vi "2-Sine Wave Chart (while loop with property nodes).vi"() -> ()   [LabVIEW 2014]
panel:
  in  "Color Box":u32(colorbox)
  in  "stop":bool
  out "Waveform Chart":dbl(graph)
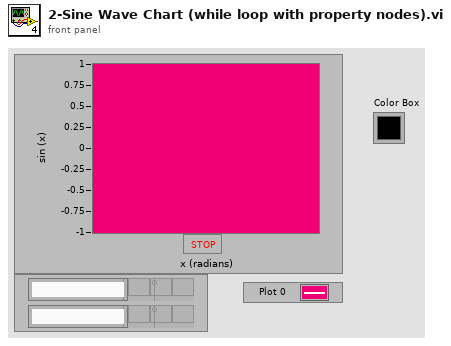
[diagram p1: front panel]
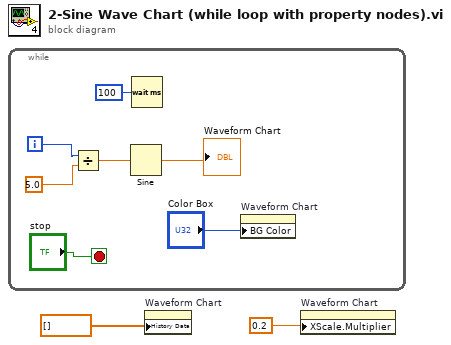
[diagram p0: block diagram]
diagram:
  n1 = while {
    i -> [w5]
    stop <- "stop" stop-if-true
    n2 = Divide(x=w5, y=5.0) -> (x/y=w7:dbl)
    n3 = Sine(x=w7) -> (sin(x)=→"Waveform Chart":dbl)
    n4 = Wait (ms)(milliseconds to wait=u32 100) -> ()  [unwired: 1 out]
    n5 = property on="Waveform Chart" class="WFChart (strict)"("BG Color"="Color Box") -> ()  [unwired: 2 in, 2 out]
  }
  n6 = property on="Waveform Chart" class="WFChart (strict)"("History Data"=dbl[] []) -> ()  [unwired: 2 in, 2 out]
  n7 = property on="Waveform Chart" class="WFChart (strict)"("XScale.Multiplier"=0.2 ("X Scale.Offset and Multiplier:Multiplier")) -> ()  [unwired: 2 in, 2 out]
